vi "Resolve Attacks.vi"(6 "Teams in":refnum<class "Team.lvclass">[](array[class]), 9 "New Map in":refnum<class "Map.lvclass">, 11 "Map in":refnum<class "Map.lvclass">) -> (1 "New Map out":refnum<class "Map.lvclass">, 4 "Teams out":refnum<class "Team.lvclass">[](array[class]))   [LabVIEW 2020, in "SquareBattle.lvlib" / "Map.lvclass"]
uses:
  Map.lvclass
  Team/Team.lvclass
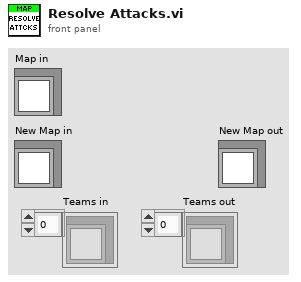
[diagram p1: front panel]
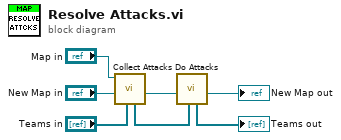
[diagram p0: block diagram]
diagram:
  n1 = call "Collect Attacks.vi"("Teams in"="Teams in", "New Map in"="New Map in", "Map in"="Map in") -> ("New Map out"=w5:refnum<class "Map.lvclass">, "Teams out"=w4:refnum<class "Team.lvclass">[])  [unwired: 7 in]
  n2 = call "Do Attacks.vi"("Teams in"=w4, "New Map in"=w5) -> ("New Map out"=→"New Map out":refnum<class "Map.lvclass">, "Teams out"=→"Teams out":refnum<class "Team.lvclass">[])  [unwired: 8 in]
